vi "refresh table.vi"(3 "Tags ref":refnum<vi>, 5 "channels ref":refnum<vi>, 7 "Mappings":refnum<vi>, 8 "error in":errorcluster, 10 "taglist":refnum<data-value>, 11 "engine configuration in":refnum<class "engine configuration.lvclass">) -> (0 "error out":errorcluster)   [LabVIEW 2013, in "PL Framework Configuration Tool.lvlib" / "Engine Mappings.lvclass"]
uses:
  Engine Mappings.lvclass
  <vilib>/NI/Module Execution Interface/Engine Configuration/engine configuration.lvclass
  <vilib>/NI/Module Execution Interface/Engine Configuration/engine configuration.lvclass/engine configuration.ctl
  <vilib>/NI/Tag Bus/tag/tag descriptor.lvclass/tag descriptor.ctl
  <vilib>/NI/Tag Bus/tag/tag descriptor.lvclass
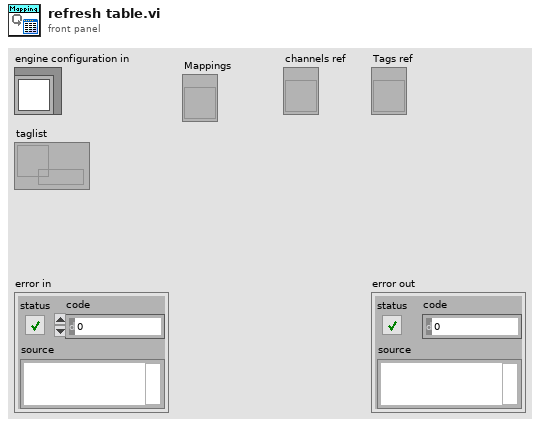
[diagram p1: front panel]
types:
  T1 = typedef "module information.ctl" = cluster{"display name":string, "instance id":string, "channels":refnum<class "TBM channel.lvclass">[]}
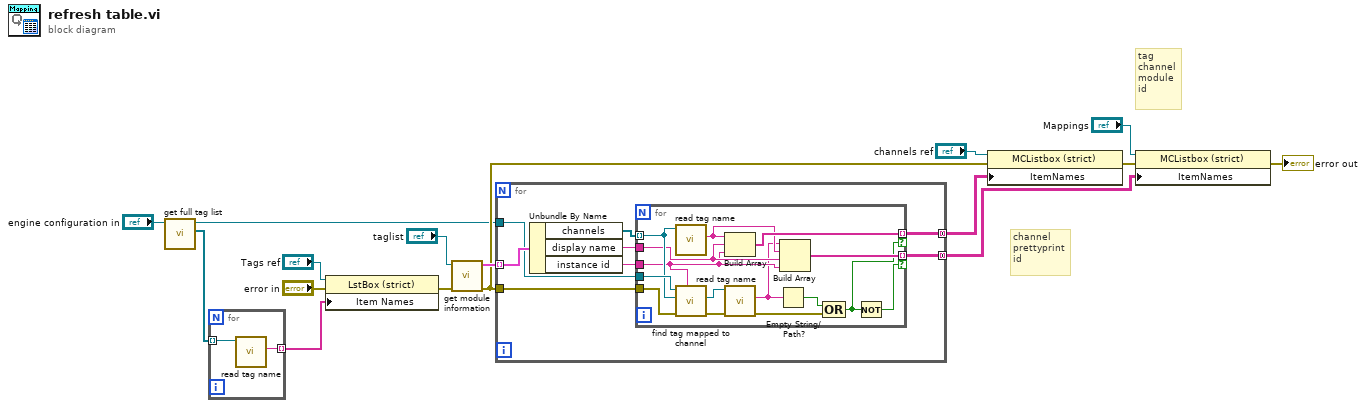
[diagram p0: block diagram]
diagram:
  # "channel\nprettyprint\nid"
  # "tag\nchannel\nmodule\nid"
  n1 = call <vilib>:"get full tag list.vi"("engine configuration in"="engine configuration in") -> ("tag list"=w16:refnum<class "tag descriptor.lvclass">[], "engine configuration out"=w3:refnum<class "engine configuration.lvclass">)  [unwired: 9 in]
  n2 = for {
    tunnel: w16 -> [w18] mode=indexing
    tunnel: [w17] -> w12 mode=indexing
    n3 = call <vilib>:"read tag name.vi"("system tag in"=w18) -> ("name"=w17:string)  [unwired: 8 in, 2 out]
  }
  n4 = property class="LstBox (strict)"(reference="Tags ref", error in="error in", "Item Names"=w12) -> (error out=w11:errorcluster)  [unwired: 1 out]
  n5 = call "get module information.vi"("error in"=w11, "engine mappings"="taglist") -> ("error out"=w4:errorcluster, "module info"=w9:T1[])  [unwired: 8 in]
  n6 = for {
    tunnel: w9 -> [w26] mode=indexing
    tunnel: w4 -> [w22]
    tunnel: w3 -> [w21]
    tunnel: [w20] -> w2 mode=concatenating
    tunnel: [w19] -> w1 mode=concatenating
    n7 = Unbundle By Name(w26) -> ("channels"=w25:refnum<class "TBM channel.lvclass">[], "display name"=w24:string, "instance id"=w23:string)
    n8 = for {
      tunnel: w25 -> [w39] mode=indexing
      tunnel: w24 -> [w33]
      tunnel: w23 -> [w32]
      tunnel: w22 -> [w40]
      tunnel: w21 -> [w41]
      tunnel: [w36] -> w20 mode=indexing if=w28
      tunnel: [w35] -> w19 mode=indexing if=w27
      n9 = call <vilib>:"read tag name.vi"("system tag in"=w39) -> ("name"=w34:string)  [unwired: 8 in, 2 out]
      n10 = call <vilib>:"find tag mapped to channel.vi"("owner"=w32, "error in"=w40, "channel"=w39, "engine configuration in"=w41) -> ("error out"=w38:errorcluster, "tag"=w37:refnum<class "tag descriptor.lvclass">)  [unwired: 5 in, 1 out]
      n11 = Build Array(w34, w33, w32) -> (w36:string[])
      n12 = call <vilib>:"read tag name.vi"("error in"=w38, "system tag in"=w37) -> ("error out"=w29:errorcluster, "name"=w31:string)  [unwired: 7 in, 1 out]
      n13 = Empty String/Path?(string/path=w31) -> (empty?=w30:bool)
      n14 = Build Array(w31, w34, w33, w32) -> (w35:string[])
      n15 = Compound Arithmetic op=OR(w30, w29) -> (w28:bool)
      n16 = Not(x=w28) -> (.not. x?=w27:bool)
    }
  }
  n17 = property class="MCListbox (strict)"(reference="channels ref", error in=w4, "ItemNames"=w2) -> (error out=w6:errorcluster)  [unwired: 1 out]
  n18 = property class="MCListbox (strict)"(reference="Mappings", error in=w6, "ItemNames"=w1) -> (error out=→"error out":errorcluster)  [unwired: 1 out]
